vi "FGVConfigFIleSemaphore.vi"(8 "error in (no error)":errorcluster, 11 "Mode":enum16{"Create", "Delete"}(ring)) -> (0 "error out":errorcluster, 3 "semaphore":T1)   [LabVIEW 2020, in "ViewableActor.lvlib"]
uses:
  ViewableActor.lvlib
panel:
  out "created new?":bool
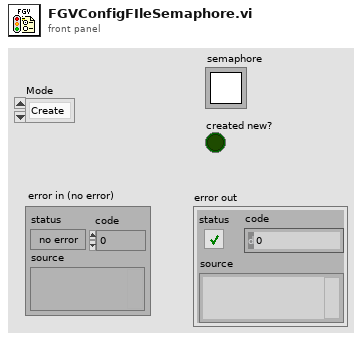
[diagram p1: front panel]
types:
  T1 = typedef "Semaphore RefNum" = refnum<k1>
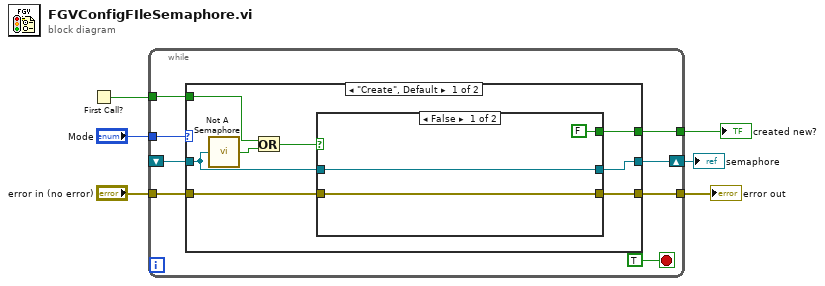
[diagram p0: block diagram]
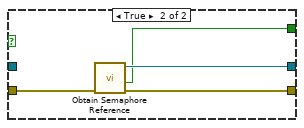
[diagram p2: hidden frame]
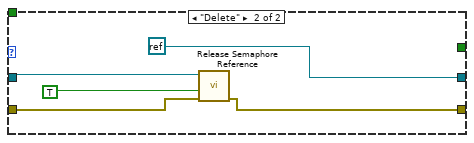
[diagram p3: hidden frame]
diagram:
  n1 = First Call?() -> (First Call?: T/F=w3:bool)
  n2 = while {
    shift-right: [w14] -> w2
    shift-left: _ -> [w13]
    tunnel: [w12] -> w5
    tunnel: "Mode" -> [w11]
    tunnel: "error in (no error)" -> [w10]
    tunnel: w3 -> [w8]
    tunnel: [w7] -> w1
    stop <- TRUE stop-if-true
    n3 = case shown="\"Create\", Default" w11 {
      tunnel: [w22 refnum<k0> refnum] -> w14
      tunnel: w13 -> [w15 w33]
      tunnel: [w21 w32] -> w12
      tunnel: w10 -> [w20 w31]
      tunnel: w8 -> [w18 _]
      tunnel: [w17 _] -> w7
      frame "Create", Default {
        n4 = call <vilib>:"Not A Semaphore.vi"("semaphore"=w15) -> ("not a semaphore"=w16:bool)
        n5 = Or(x=w18, y=w16) -> (x .or. y?=w19:bool)
        n6 = case shown="False" w19 {
          tunnel: [w25 w27] -> w22
          tunnel: w15 -> [w25 _]
          tunnel: [w24 w28] -> w21
          tunnel: w20 -> [w24 w29]
          tunnel: [FALSE ("created new") w26] -> w17
          frame False {
          }
          frame True {
            n7 = call <vilib>:"Obtain Semaphore Reference.vi"("error in (no error)"=w29) -> ("error out"=w28:errorcluster, "created new"=w26:bool, "semaphore"=w27:T1)  [unwired: 4 in]
          }
        }
      }
      frame "Delete" {
        n8 = call <vilib>:"Release Semaphore Reference.vi"("error in (no error)"=w31, "force destroy? (F)"=TRUE, "semaphore"=w33) -> ("error out"=w32:errorcluster)  [unwired: 7 in, 1 out]
      }
    }
  }
  "error out" <- w5
  "semaphore" <- w2
  "created new?" <- w1
